vi "Add Item.vi"(7 "Action":T1, 8 "error in (no error)":errorcluster, 11 "Listbox Refs in":T2 {"Section Ref" format="%.0x"}) -> (0 "error out":errorcluster, 3 "Listbox Refs out":T2 {"Section Ref" format="%.0x"})   [LabVIEW 2016, in "FPGA Addon System Explorer.lvlib"]
uses:
  FPGA Addon System Explorer.lvlib
  Listbox Cluster.ctl
  <vilib>/NI Veristand/Custom Device API/Custom Device Item Ref.ctl
  FPGA-Resource-Manager-APIs/Source/Shared/Types/Channel Type.ctl
  <vilib>/NI Veristand/Custom Device API/Custom Device Channel.ctl
  <vilib>/NI Veristand/Custom Device API/Custom Device Channel Type.ctl
  FPGA/Speciality IO/Types/PWM.Measure.Analog.Settings.ctl
  FPGA/Speciality IO/Types/PWM.Generate.Digital.Settings.ctl
  FPGA/Speciality IO/Types/PWM.Generate.Digital.Convert.Settings.ctl
  FPGA/Speciality IO/Types/Sine.Generate.Settings.ctl
  FPGA/Speciality IO/Types/Sine.Generate.Convert.Settings.ctl
  FPGA/Speciality IO/Types/PWM.Measure.Digital.Settings.ctl
  FPGA/Speciality IO/Types/PWM.Measure.Analog.Result.ctl
  FPGA/Speciality IO/Types/PWM.Measure.Digital.Result.ctl
  FPGA-Resource-Manager-APIs/Source/System Definition/API/Server-Specific/Resource Groups/get fpga resources compatible with FPGA Addon CD group.vi
  Shared/Constants.vi
  RegMap to Register Information.vi
  FPGA-Resource-Manager-APIs/Source/System Definition/API/FPGA Resource Discovery/get FPGA resources for this FPGA Addon CD.vi
  FPGA-Resource-Manager-APIs/Source/Shared/find Relative VS Ref.vi
  <vilib>/NI Veristand/Custom Device API/NI VeriStand - Get Item Data.vi
  <vilib>/NI VeriStand/Custom Device API/Custom Device API.lvlib
  Shared/FPGA Addon Shared.lvlib
  FPGA/Speciality IO/Speciality FPGA IO.lvlib
  FPGA-Resource-Manager-APIs/Source/System Definition/FPGA RM System Definition API.lvlib
  FPGA-Resource-Manager-APIs/Source/Shared/FPGA RM Shared API.lvlib
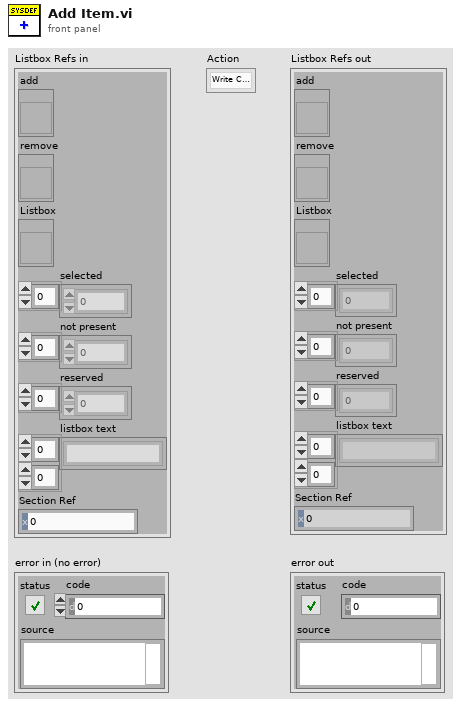
[diagram p1: front panel]
types:
  T1 = typedef "FPGA RM Shared API.lvlib/Channel Type.ctl" = enum16{"Write Channel", "Read Channel", "Write Waveform", "Read Waveform"}
  T2 = typedef "FPGA Addon System Explorer.lvlib/Listbox Cluster.ctl" = cluster{"add":refnum<vi>, "remove":refnum<vi>, "Listbox":refnum<vi>, "selected":i32[], "not present":i32[], "reserved":i32[], "listbox text":string[][], "Section Ref":T3}
  T3 = typedef "Custom Device API.lvlib/Custom Device Item Ref.ctl" = u64
  T4 = typedef "Custom Device API.lvlib/Custom Device Channel.ctl" = cluster{"Type":T5, "Units":string, "Default Value":dbl, "Faultable":bool, "Scalable":bool}
  T5 = typedef "Custom Device API.lvlib/Custom Device Channel Type.ctl" = enum16{"Input", "Output"}
  T6 = typedef "Speciality FPGA IO.lvlib/PWM.Measure.Analog.Settings.ctl" = cluster{"ACTIVE EDGE":bool, "TIMEOUT":u32, "THRESHOLD":fxp<+/-,32,8>}
  T7 = typedef "Speciality FPGA IO.lvlib/PWM.Generate.Digital.Convert.Settings.ctl" = cluster{"ACTIVE EDGE":bool, "FREQ":sgl, "DC":sgl}
  T8 = typedef "Speciality FPGA IO.lvlib/PWM.Generate.Digital.Settings.ctl" = cluster{"ACTIVE EDGE":bool, "ACTIVE TICKS":u32, "INACTIVE TICKS":u32}
  T9 = typedef "Speciality FPGA IO.lvlib/Sine.Generate.Convert.Settings.ctl" = cluster{"AMP":sgl, "OFFSET":sgl, "FREQ":sgl}
  T10 = typedef "Speciality FPGA IO.lvlib/Sine.Generate.Settings.ctl" = cluster{"AMP":fxp<+/-,32,8>, "OFFSET":fxp<+/-,32,8>, "PERIODS/TICKS":fxp<+,32,0>}
  T11 = typedef "Speciality FPGA IO.lvlib/PWM.Measure.Analog.Result.ctl" = cluster{"FREQ":sgl, "PERIOD":sgl, "DC":sgl, "ACTIVE TIME":sgl, "ACTIVE VOLTAGE":sgl, "INACTIVE VOLTAGE":sgl}
  T12 = typedef "Speciality FPGA IO.lvlib/PWM.Measure.Digital.Result.ctl" = cluster{"FREQ":sgl, "PERIOD":sgl, "DC":sgl, "ACTIVE TIME":sgl}
  T13 = typedef "FPGA RM Shared API.lvlib/Register Information.ctl" = cluster{"Name":string, "Data Type":T14, "Default Value":variant}
  T14 = typedef "FPGA RM Shared API.lvlib/Data Type.ctl" = enum8{"<Null>", "I8", "I16", "I32", "I64", "U8", "U16", "U32", "U64", "SGL", "Boolean", "Analog PWM In Settings", "Analog PWM In", "Digital PWM In Settings", "Digital PWM In", "Digital PWM Out", "Sine Out", "FXP+/-24.5", "FXP+/-16.5", "FXP+/-32.8", "FXP+/-64.32", "FXP+/-16.7", "FXP+/-20.5"}
  T15 = typedef "Speciality FPGA IO.lvlib/PWM.Measure.Digital.Settings.ctl" = cluster{"ACTIVE EDGE":bool, "TIMEOUT":u32}
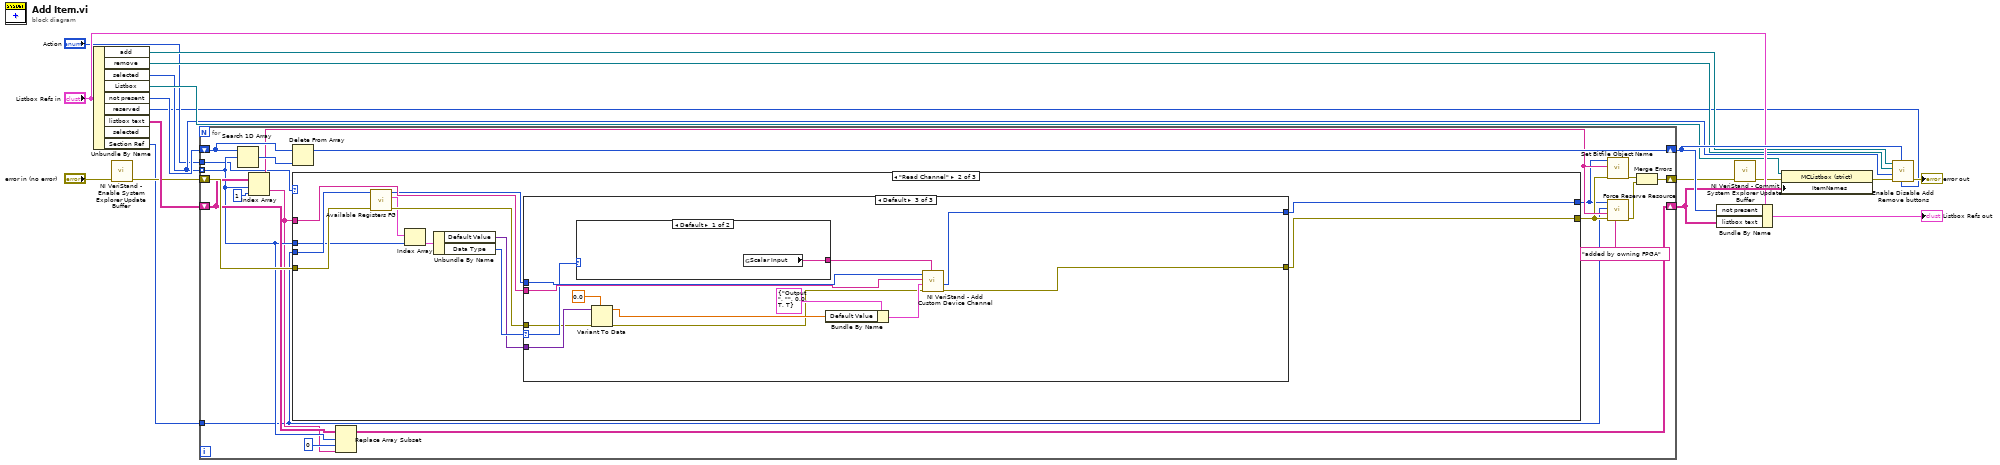
[diagram p0: block diagram]
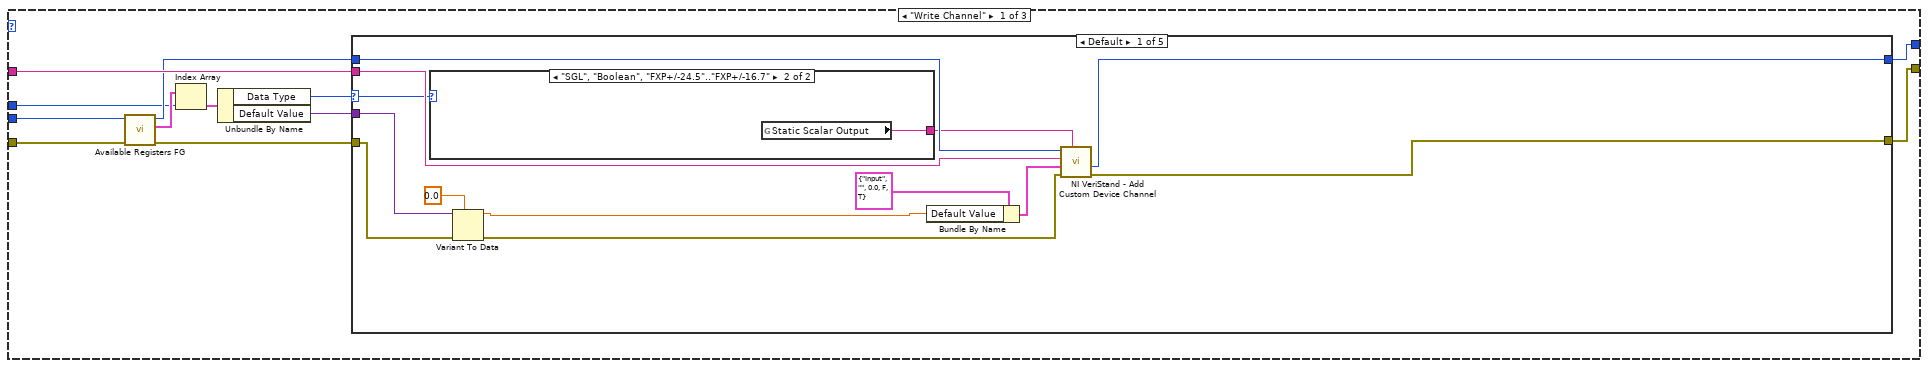
[diagram p2: hidden frame]
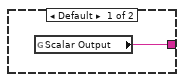
[diagram p3: hidden frame]
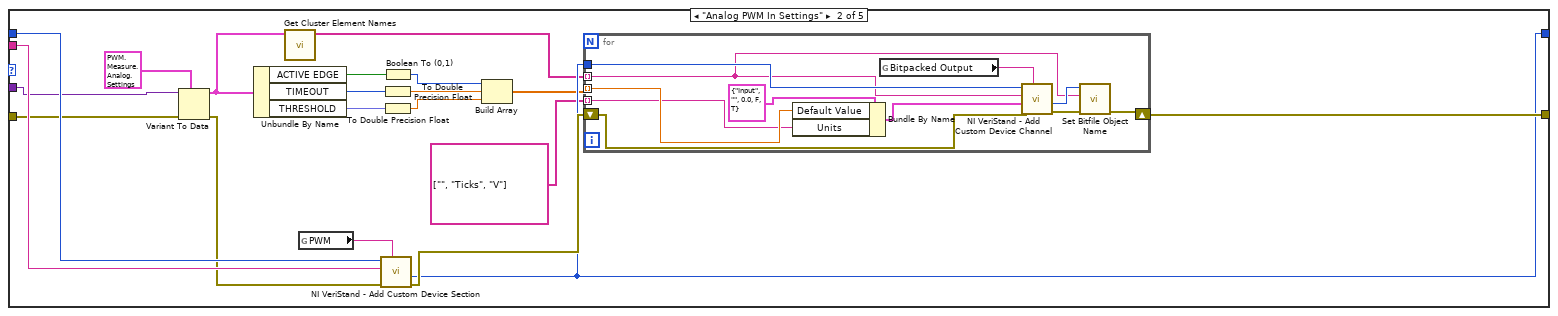
[diagram p4: hidden frame]
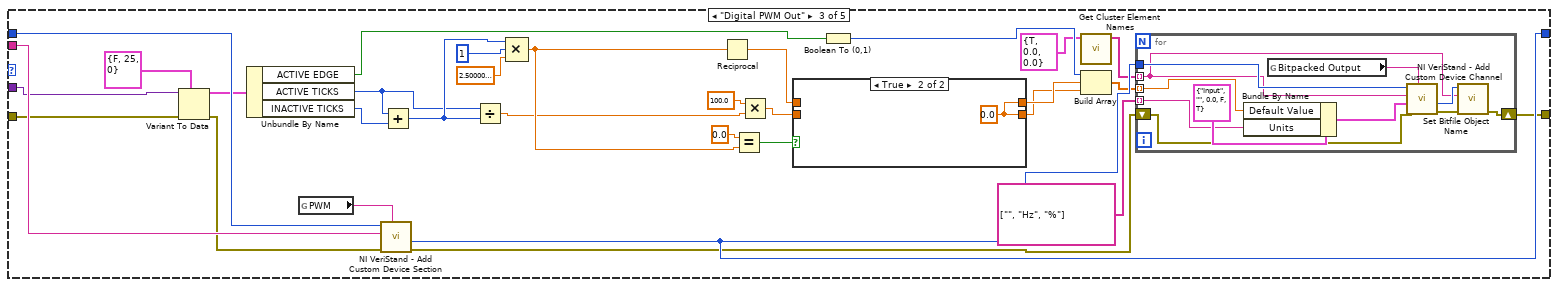
[diagram p5: hidden frame]
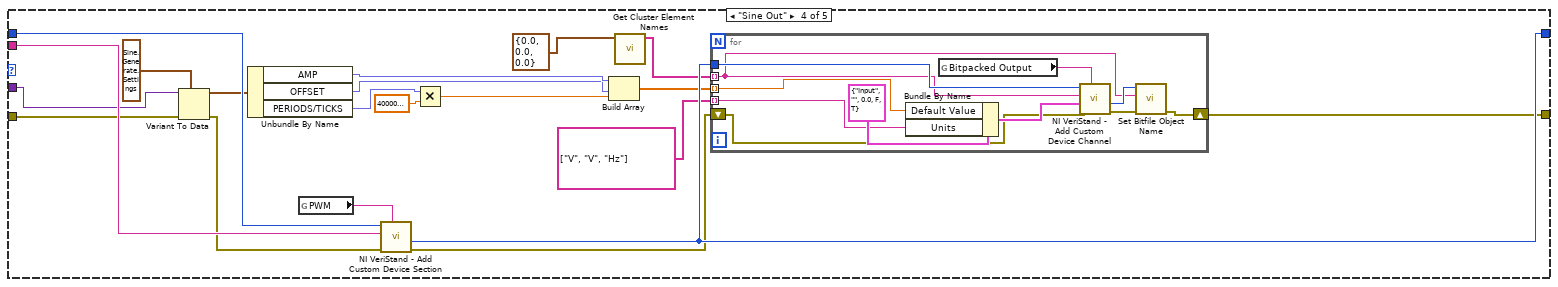
[diagram p7: hidden frame]
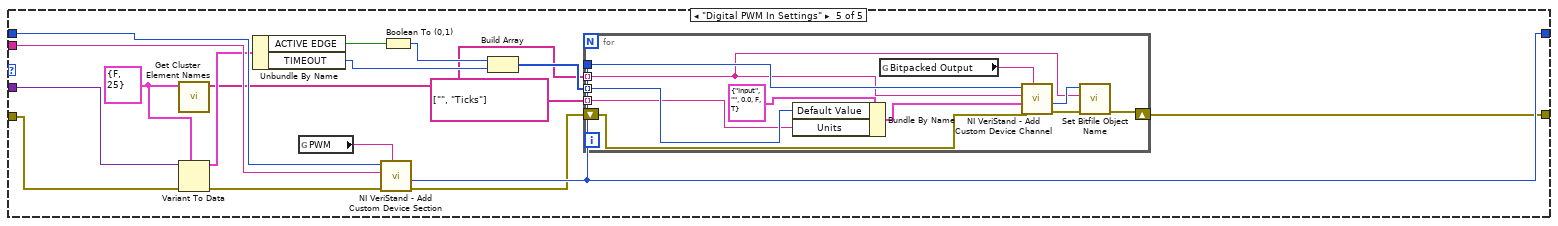
[diagram p8: hidden frame]
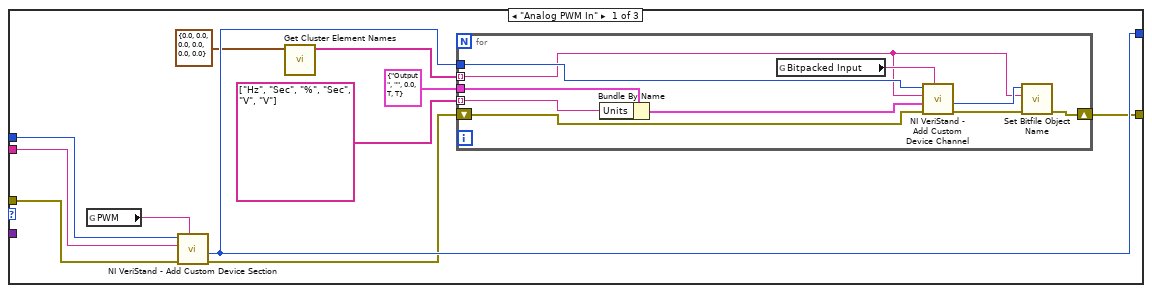
[diagram p9: hidden frame]
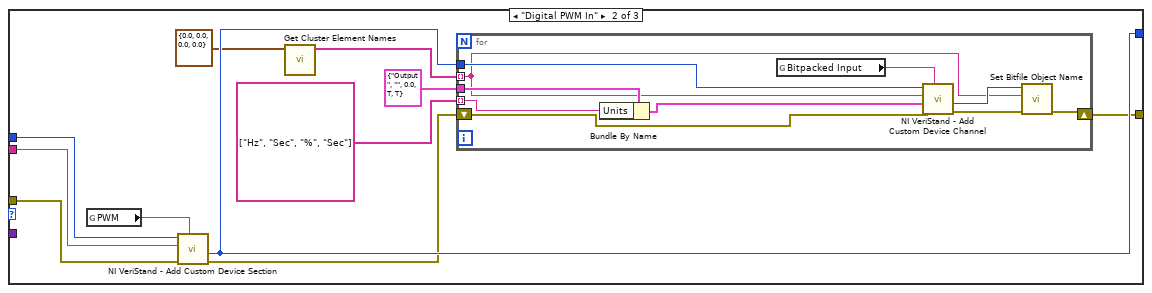
[diagram p10: hidden frame]
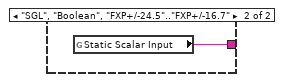
[diagram p11: hidden frame]
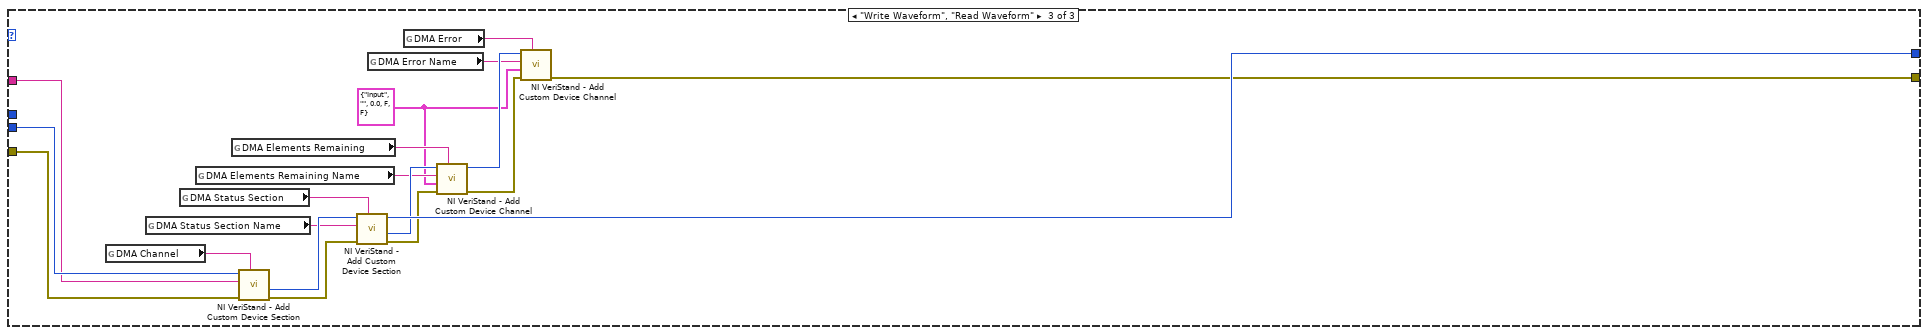
[diagram p12: hidden frame]
diagram:
  n1 = Unbundle By Name("Listbox Refs in") -> ("add"=w11:refnum<vi>, "remove"=w12:refnum<vi>, "selected"=w4:i32[], "Listbox"=w5:refnum<vi>, "not present"=w10:i32[], "reserved"=w1:i32[], "listbox text"=w18:string[][], "Section Ref"=w6:T3)  [unwired: 1 out]
  n2 = call <vilib>:"NI VeriStand - Enable System Explorer Update Buffer.vi"("error in (no error)"="error in (no error)") -> ("error out"=w9:errorcluster)  [unwired: 10 in]
  n3 = for {
    tunnel: w6 -> [w22]
    shift-right: [w25] -> w7
    shift-left: w9 -> [w37]
    tunnel: w4 -> [w29] mode=indexing
    shift-right: [w34] -> w16
    shift-left: w18 -> [w35]
    shift-right: [w30] -> w17
    shift-left: w10 -> [w32]
    tunnel: "Action" -> [w21]
    n4 = Search 1D Array(1D array=w32, element=w29) -> (index of element=w31:i32)  [unwired: 1 in]
    n5 = Index Array(array=w35, index (row)=w29, index (col)=1 ("disabled index (col)")) -> (element=w27:string)
    n6 = Delete From Array(array=w32, index=w31) -> (array with subset deleted=w30:i32[])  [unwired: 1 in, 1 out]
    n7 = case shown="\"Read Channel\"" w21 {
      tunnel: w37 -> [w44 w207 w286]
      tunnel: [w49 w211 w277] -> w26
      tunnel: w22 -> [w43 w208 w287]
      tunnel: w27 -> [w48 w210 w271]
      tunnel: [w47 w209 w282] -> w23
      tunnel: w29 -> [w40 w203 _]
      frame "Write Channel" {
        n8 = call "Available Registers FG.vi"("error in (no error)"=w44, "Item Ref"=w43) -> ("error out"=w41:errorcluster, "Available Registers"=w46:T13[], "Item Ref out"=w42:T3)  [unwired: 7 in]
        n9 = Index Array(array=w46, index=w40) -> (element=w45:T13)
        n10 = Unbundle By Name(w45) -> ("Data Type"=w38:T14, "Default Value"=w39:variant)
        n11 = case shown="Default" w38 {
          selector: w38 -> [w55 _ _ _ _]
          tunnel: [w62 w78 w120 w154 w182] -> w49
          tunnel: w48 -> [w61 w84 w126 w160 w188]
          tunnel: [w60 w77 w122 w156 w184] -> w47
          tunnel: w42 -> [w59 w83 w125 w159 w187]
          tunnel: w41 -> [w51 w81 w123 w157 w185]
          tunnel: w39 -> [w54 w82 w124 w158 w186]
          frame Default {
            n12 = case shown="\"SGL\", \"Boolean\", \"FXP+/-24.5\"..\"FXP+/-16.7\"" w55 {
              tunnel: [w63 w64] -> w58
              frame Default {
                n13 = global read "Constants.vi" "Scalar Output"() -> (w63:string)
              }
              frame "SGL", "Boolean", "FXP+/-24.5".."FXP+/-16.7" {
                n14 = global read "Constants.vi" "Static Scalar Output"() -> (w64:string)
              }
            }
            n15 = Variant To Data(error in=w51, type=0.0 ("Default Value"), Variant=w54) -> (data=w52:dbl, error out=w50:errorcluster)
            n16 = Bundle By Name(cluster=T4 {"Type"=enum."Input", "Units"="", "Default Value"=0.0, "Faultable"=FALSE, "Scalable"=TRUE} ("Channel"), "Default Value"=w52) -> (w56:T4)
            n17 = call <vilib>:"NI VeriStand - Add Custom Device Channel.vi"("GUID (Default Channel)"=w58, "error in (no error)"=w50, "Channel"=w56, "Channel Name"=w61, "Parent Ref in"=w59) -> ("error out"=w62:errorcluster, "Channel Ref"=w60:T3)  [unwired: 3 in, 2 out]
          }
          frame "Analog PWM In Settings" {
            n18 = Variant To Data(error in=w81, type=T6 {"ACTIVE EDGE"=FALSE, "TIMEOUT"=1000000000, "THRESHOLD"=25.0} ("Channel.Settings"), Variant=w82) -> (data=w66:T6, error out=w67:errorcluster)
            n19 = Unbundle By Name(w66) -> ("ACTIVE EDGE"=w72:bool, "TIMEOUT"=w76:u32, "THRESHOLD"=w71:fxp<+/-,32,8>)
            n20 = call "Get Cluster Element Names.vi"("Cluster"=w66) -> ("Channels"=w65:string[])  [unwired: 10 in]
            n21 = global read "Constants.vi" "PWM"() -> (w68:string)
            n22 = call <vilib>:"NI VeriStand - Add Custom Device Section.vi"("GUID (Default Section)"=w68, "error in (no error)"=w67, "Section Name"=w84, "Parent Ref in"=w83) -> ("error out"=w79:errorcluster, "Section Ptr"=w77:T3)  [unwired: 4 in, 2 out]
            n23 = Boolean To (0,1)(Boolean=w72) -> (0, 1=w70:i16)
            n24 = To Double Precision Float(number=w76) -> (double precision float=w74:dbl)
            n25 = To Double Precision Float(number=w71) -> (double precision float=w69:dbl)
            n26 = Build Array(w70, w74, w69) -> (w75:dbl[])
            n27 = for {
              tunnel: w77 -> [w93]
              shift-right: [w86] -> w78
              shift-left: w79 -> [w92]
              tunnel: w75 -> [w90] mode=indexing
              tunnel: string[] ["", "Ticks", "V"] -> [w89] mode=indexing
              tunnel: w65 -> [w85] mode=indexing
              n28 = Bundle By Name(cluster=T4 {"Type"=enum."Input", "Units"="", "Default Value"=0.0, "Faultable"=FALSE, "Scalable"=TRUE} ("Channel"), "Default Value"=w90, "Units"=w89) -> (w94:T4)
              n29 = global read "Constants.vi" "Bitpacked Output"() -> (w91:string)
              n30 = call <vilib>:"NI VeriStand - Add Custom Device Channel.vi"("GUID (Default Channel)"=w91, "error in (no error)"=w92, "Channel"=w94, "Channel Name"=w85, "Parent Ref in"=w93) -> ("error out"=w87:errorcluster, "Channel Ref"=w88:T3)  [unwired: 3 in, 2 out]
              n31 = call "Set Bitfile Object Name.vi"("error in (no error)"=w87, "Name"=w85, "Channel Ref"=w88) -> ("error out"=w86:errorcluster)  [unwired: 8 in]
            }
          }
          frame "Digital PWM Out" {
            n32 = Variant To Data(error in=w123, type=T8 {"ACTIVE EDGE"=FALSE, "ACTIVE TICKS"=25, "INACTIVE TICKS"=0} ("Channel.Settings"), Variant=w124) -> (data=w119:T8, error out=w112:errorcluster)
            n33 = Unbundle By Name(w119) -> ("ACTIVE EDGE"=w118:bool, "ACTIVE TICKS"=w103:u32, "INACTIVE TICKS"=w102:u32)
            n34 = global read "Constants.vi" "PWM"() -> (w115:string)
            n35 = call <vilib>:"NI VeriStand - Add Custom Device Section.vi"("GUID (Default Section)"=w115, "error in (no error)"=w112, "Section Name"=w126, "Parent Ref in"=w125) -> ("error out"=w121:errorcluster, "Section Ptr"=w122:T3)  [unwired: 4 in, 2 out]
            n36 = Add(x=w103, y=w102) -> (x+y=w109:u32)
            n37 = Divide(x=w103, y=w109) -> (x/y=w105:dbl)
            n38 = Compound Arithmetic op=MULTIPLY(w109, u32 1 ("value"), 2.5000000292152436e-08 ("y")) -> (w110:dbl)
            n39 = Reciprocal(x=w110) -> (1/x=w99:dbl)
            n40 = Equal?(x=0.0, y=w110) -> (x = y?=w101:bool)
            n41 = Multiply(x=100.0, y=w105) -> (x*y=w97:dbl)
            n42 = case shown="True" w101 {
              tunnel: [w128 w129] -> w100
              tunnel: w99 -> [w128 _]
              tunnel: [w127 w129] -> w98
              tunnel: w97 -> [w127 _]
              frame False {
              }
              frame True {
                w129 = 0.0
              }
            }
            n43 = Boolean To (0,1)(Boolean=w118) -> (0, 1=w117:i16)
            n44 = call "Get Cluster Element Names.vi"("Cluster"=T7 {"ACTIVE EDGE"=TRUE, "FREQ"=0.0, "DC"=0.0} ("Settings")) -> ("Channels"=w113:string[])  [unwired: 10 in]
            n45 = Build Array(w117, w100, w98) -> (w116:dbl[])
            n46 = for {
              tunnel: w122 -> [w138]
              shift-right: [w131] -> w120
              shift-left: w121 -> [w137]
              tunnel: w116 -> [w135] mode=indexing
              tunnel: w113 -> [w130] mode=indexing
              tunnel: string[] ["", "Hz", "%"] -> [w134] mode=indexing
              n47 = Bundle By Name(cluster=T4 {"Type"=enum."Input", "Units"="", "Default Value"=0.0, "Faultable"=FALSE, "Scalable"=TRUE} ("Channel"), "Default Value"=w135, "Units"=w134) -> (w139:T4)
              n48 = global read "Constants.vi" "Bitpacked Output"() -> (w136:string)
              n49 = call <vilib>:"NI VeriStand - Add Custom Device Channel.vi"("GUID (Default Channel)"=w136, "error in (no error)"=w137, "Channel"=w139, "Channel Name"=w130, "Parent Ref in"=w138) -> ("error out"=w132:errorcluster, "Channel Ref"=w133:T3)  [unwired: 3 in, 2 out]
              n50 = call "Set Bitfile Object Name.vi"("error in (no error)"=w132, "Name"=w130, "Channel Ref"=w133) -> ("error out"=w131:errorcluster)  [unwired: 8 in]
            }
          }
          frame "Sine Out" {
            n51 = Variant To Data(error in=w157, type=T10 {"AMP"=0.0, "OFFSET"=0.0, "PERIODS/TICKS"=0.0} ("Settings"), Variant=w158) -> (data=w153:T10, error out=w148:errorcluster)
            n52 = Unbundle By Name(w153) -> ("AMP"=w146:fxp<+/-,32,8>, "OFFSET"=w145:fxp<+/-,32,8>, "PERIODS/TICKS"=w144:fxp<+,32,0>)
            n53 = global read "Constants.vi" "PWM"() -> (w151:string)
            n54 = call <vilib>:"NI VeriStand - Add Custom Device Section.vi"("GUID (Default Section)"=w151, "error in (no error)"=w148, "Section Name"=w160, "Parent Ref in"=w159) -> ("error out"=w155:errorcluster, "Section Ptr"=w156:T3)  [unwired: 4 in, 2 out]
            n55 = Multiply(x=w144, y=sgl 40000000.0) -> (x*y=w142:sgl)
            n56 = Build Array(w146, w145, w142) -> (w152:sgl[])
            n57 = call "Get Cluster Element Names.vi"("Cluster"=T9 {"AMP"=0.0, "OFFSET"=0.0, "FREQ"=0.0} ("Settings")) -> ("Channels"=w149:string[])  [unwired: 10 in]
            n58 = for {
              tunnel: w156 -> [w169]
              shift-right: [w162] -> w154
              shift-left: w155 -> [w168]
              tunnel: w152 -> [w166] mode=indexing
              tunnel: w149 -> [w161] mode=indexing
              tunnel: string[] ["V", "V", "Hz"] -> [w165] mode=indexing
              n59 = Bundle By Name(cluster=T4 {"Type"=enum."Input", "Units"="", "Default Value"=0.0, "Faultable"=FALSE, "Scalable"=TRUE} ("Channel"), "Default Value"=w166, "Units"=w165) -> (w170:T4)
              n60 = global read "Constants.vi" "Bitpacked Output"() -> (w167:string)
              n61 = call <vilib>:"NI VeriStand - Add Custom Device Channel.vi"("GUID (Default Channel)"=w167, "error in (no error)"=w168, "Channel"=w170, "Channel Name"=w161, "Parent Ref in"=w169) -> ("error out"=w163:errorcluster, "Channel Ref"=w164:T3)  [unwired: 3 in, 2 out]
              n62 = call "Set Bitfile Object Name.vi"("error in (no error)"=w163, "Name"=w161, "Channel Ref"=w164) -> ("error out"=w162:errorcluster)  [unwired: 8 in]
            }
          }
          frame "Digital PWM In Settings" {
            w175 = T15 {"ACTIVE EDGE"=FALSE, "TIMEOUT"=25} ("Channel.Settings")
            n63 = call "Get Cluster Element Names.vi"("Cluster"=w175) -> ("Channels"=w174:string[])  [unwired: 10 in]
            n64 = Variant To Data(error in=w185, type=w175, Variant=w186) -> (data=w178:T15, error out=w173:errorcluster)
            n65 = Unbundle By Name(w178) -> ("ACTIVE EDGE"=w181:bool, "TIMEOUT"=w180:u32)
            n66 = global read "Constants.vi" "PWM"() -> (w176:string)
            n67 = call <vilib>:"NI VeriStand - Add Custom Device Section.vi"("GUID (Default Section)"=w176, "error in (no error)"=w173, "Section Name"=w188, "Parent Ref in"=w187) -> ("error out"=w183:errorcluster, "Section Ptr"=w184:T3)  [unwired: 4 in, 2 out]
            n68 = Boolean To (0,1)(Boolean=w181) -> (0, 1=w179:i16)
            n69 = Build Array(w179, w180) -> (w177:u32[])
            n70 = for {
              tunnel: w184 -> [w197]
              shift-right: [w191] -> w182
              shift-left: w183 -> [w196]
              tunnel: w177 -> [w194] mode=indexing
              tunnel: w174 -> [w189] mode=indexing
              tunnel: string[] ["", "Ticks"] -> [w193] mode=indexing
              n71 = Bundle By Name(cluster=T4 {"Type"=enum."Input", "Units"="", "Default Value"=0.0, "Faultable"=FALSE, "Scalable"=TRUE} ("Channel"), "Default Value"=w194, "Units"=w193) -> (w198:T4)
              n72 = global read "Constants.vi" "Bitpacked Output"() -> (w195:string)
              n73 = call <vilib>:"NI VeriStand - Add Custom Device Channel.vi"("GUID (Default Channel)"=w195, "error in (no error)"=w196, "Channel"=w198, "Channel Name"=w189, "Parent Ref in"=w197) -> ("error out"=w192:errorcluster, "Channel Ref"=w190:T3)  [unwired: 3 in, 2 out]
              n74 = call "Set Bitfile Object Name.vi"("error in (no error)"=w192, "Name"=w189, "Channel Ref"=w190) -> ("error out"=w191:errorcluster)  [unwired: 8 in]
            }
          }
        }
      }
      frame "Read Channel" {
        n75 = call "Available Registers FG.vi"("error in (no error)"=w207, "Item Ref"=w208) -> ("error out"=w206:errorcluster, "Available Registers"=w204:T13[], "Item Ref out"=w205:T3)  [unwired: 7 in]
        n76 = Index Array(array=w204, index=w203) -> (element=w202:T13)
        n77 = Unbundle By Name(w202) -> ("Default Value"=w200:variant, "Data Type"=w201:T14)
        n78 = case shown="Default" w201 {
          selector: w201 -> [_ _ w259]
          tunnel: [w217 w238 w266] -> w211
          tunnel: w210 -> [w220 w241 w265]
          tunnel: [w218 w239 w264] -> w209
          tunnel: w206 -> [w222 w243 w255]
          tunnel: w205 -> [w221 w242 w263]
          tunnel: w200 -> [_ _ w258]
          frame "Analog PWM In" {
            n79 = global read "Constants.vi" "PWM"() -> (w215:string)
            n80 = call <vilib>:"NI VeriStand - Add Custom Device Section.vi"("GUID (Default Section)"=w215, "error in (no error)"=w222, "Section Name"=w220, "Parent Ref in"=w221) -> ("error out"=w212:errorcluster, "Section Ptr"=w218:T3)  [unwired: 4 in, 2 out]
            n81 = call "Get Cluster Element Names.vi"("Cluster"=T11 {"FREQ"=0.0, "PERIOD"=0.0, "DC"=0.0, "ACTIVE TIME"=0.0, "ACTIVE VOLTAGE"=0.0, "INACTIVE VOLTAGE"=0.0} ("Analyzed")) -> ("Channels"=w213:string[])  [unwired: 10 in]
            n82 = for {
              tunnel: T4 {"Type"=enum."Output", "Units"="", "Default Value"=0.0, "Faultable"=TRUE, "Scalable"=TRUE} ("Channel") -> [w229]
              tunnel: w218 -> [w232]
              shift-right: [w224] -> w217
              shift-left: w212 -> [w231]
              tunnel: string[] ["Hz", "Sec", "%", "Sec", "V", "V"] -> [w227] mode=indexing
              tunnel: w213 -> [w223] mode=indexing
              n83 = Bundle By Name(cluster=w229, "Units"=w227) -> (w228:T4)
              n84 = global read "Constants.vi" "Bitpacked Input"() -> (w230:string)
              n85 = call <vilib>:"NI VeriStand - Add Custom Device Channel.vi"("GUID (Default Channel)"=w230, "error in (no error)"=w231, "Channel"=w228, "Channel Name"=w223, "Parent Ref in"=w232) -> ("error out"=w225:errorcluster, "Channel Ref"=w226:T3)  [unwired: 3 in, 2 out]
              n86 = call "Set Bitfile Object Name.vi"("error in (no error)"=w225, "Name"=w223, "Channel Ref"=w226) -> ("error out"=w224:errorcluster)  [unwired: 8 in]
            }
          }
          frame "Digital PWM In" {
            n87 = global read "Constants.vi" "PWM"() -> (w236:string)
            n88 = call <vilib>:"NI VeriStand - Add Custom Device Section.vi"("GUID (Default Section)"=w236, "error in (no error)"=w243, "Section Name"=w241, "Parent Ref in"=w242) -> ("error out"=w233:errorcluster, "Section Ptr"=w239:T3)  [unwired: 4 in, 2 out]
            n89 = call "Get Cluster Element Names.vi"("Cluster"=T12 {"FREQ"=0.0, "PERIOD"=0.0, "DC"=0.0, "ACTIVE TIME"=0.0} ("Analyzed")) -> ("Channels"=w234:string[])  [unwired: 10 in]
            n90 = for {
              tunnel: T4 {"Type"=enum."Output", "Units"="", "Default Value"=0.0, "Faultable"=TRUE, "Scalable"=TRUE} ("Channel") -> [w253]
              tunnel: w239 -> [w252]
              shift-right: [w244] -> w238
              shift-left: w233 -> [w251]
              tunnel: string[] ["Hz", "Sec", "%", "Sec"] -> [w248] mode=indexing
              tunnel: w234 -> [w246] mode=indexing
              n91 = Bundle By Name(cluster=w253, "Units"=w248) -> (w249:T4)
              n92 = global read "Constants.vi" "Bitpacked Input"() -> (w250:string)
              n93 = call <vilib>:"NI VeriStand - Add Custom Device Channel.vi"("GUID (Default Channel)"=w250, "error in (no error)"=w251, "Channel"=w249, "Channel Name"=w246, "Parent Ref in"=w252) -> ("error out"=w245:errorcluster, "Channel Ref"=w247:T3)  [unwired: 3 in, 2 out]
              n94 = call "Set Bitfile Object Name.vi"("error in (no error)"=w245, "Name"=w246, "Channel Ref"=w247) -> ("error out"=w244:errorcluster)  [unwired: 8 in]
            }
          }
          frame Default {
            n95 = case shown="Default" w259 {
              tunnel: [w267 w268] -> w262
              frame Default {
                n96 = global read "Constants.vi" "Scalar Input"() -> (w267:string)
              }
              frame "SGL", "Boolean", "FXP+/-24.5".."FXP+/-16.7" {
                n97 = global read "Constants.vi" "Static Scalar Input"() -> (w268:string)
              }
            }
            n98 = Variant To Data(error in=w255, type=0.0, Variant=w258) -> (data=w256:dbl, error out=w254:errorcluster)
            n99 = Bundle By Name(cluster=T4 {"Type"=enum."Output", "Units"="", "Default Value"=0.0, "Faultable"=TRUE, "Scalable"=TRUE} ("Channel"), "Default Value"=w256) -> (w260:T4)
            n100 = call <vilib>:"NI VeriStand - Add Custom Device Channel.vi"("GUID (Default Channel)"=w262, "error in (no error)"=w254, "Channel"=w260, "Channel Name"=w265, "Parent Ref in"=w263) -> ("error out"=w266:errorcluster, "Channel Ref"=w264:T3)  [unwired: 3 in, 2 out]
          }
        }
      }
      frame "Write Waveform", "Read Waveform" {
        w272 = T4 {"Type"=enum."Input", "Units"="", "Default Value"=0.0, "Faultable"=FALSE, "Scalable"=FALSE} ("Channel")
        n101 = global read "Constants.vi" "DMA Channel"() -> (w285:string)
        n102 = global read "Constants.vi" "DMA Status Section Name"() -> (w270:string)
        n103 = global read "Constants.vi" "DMA Status Section"() -> (w269:string)
        n104 = global read "Constants.vi" "DMA Elements Remaining Name"() -> (w275:string)
        n105 = global read "Constants.vi" "DMA Elements Remaining"() -> (w276:string)
        n106 = call <vilib>:"NI VeriStand - Add Custom Device Section.vi"("GUID (Default Section)"=w285, "error in (no error)"=w286, "Section Name"=w271, "Parent Ref in"=w287) -> ("error out"=w284:errorcluster, "Section Ptr"=w283:T3)  [unwired: 4 in, 2 out]
        n107 = call <vilib>:"NI VeriStand - Add Custom Device Section.vi"("GUID (Default Section)"=w269, "error in (no error)"=w284, "Section Name"=w270, "Parent Ref in"=w283) -> ("error out"=w278:errorcluster, "Section Ptr"=w279:T3, "Parent Ref out"=w282:T3)  [unwired: 4 in, 1 out]
        n108 = global read "Constants.vi" "DMA Error Name"() -> (w274:string)
        n109 = global read "Constants.vi" "DMA Error"() -> (w273:string)
        n110 = call <vilib>:"NI VeriStand - Add Custom Device Channel.vi"("GUID (Default Channel)"=w276, "error in (no error)"=w278, "Channel"=w272, "Channel Name"=w275, "Parent Ref in"=w279) -> ("error out"=w280:errorcluster, "Parent Ref out"=w281:T3)  [unwired: 3 in, 2 out]
        n111 = call <vilib>:"NI VeriStand - Add Custom Device Channel.vi"("GUID (Default Channel)"=w273, "error in (no error)"=w280, "Channel"=w272, "Channel Name"=w274, "Parent Ref in"=w281) -> ("error out"=w277:errorcluster)  [unwired: 3 in, 3 out]
      }
    }
    n112 = Replace Array Subset(array=w35, new element=w27, index (row)=w29, index (col)=0 ("disabled index (col)")) -> (w34:string[][])
    n113 = call "Set Bitfile Object Name.vi"("error in (no error)"=w26, "Name"=w27, "Channel Ref"=w23) -> ("error out"=w28:errorcluster)  [unwired: 8 in]
    n114 = call "Force Reserve Resource.vi"("notes"="added by owning FPGA", "error in (no error)"=w26, "Name in bitfile"=w27, "Client Node Ref"=w22, "Item Ref in"=w23) -> ("error out"=w24:errorcluster)  [unwired: 5 in, 1 out]
    n115 = Merge Errors(w28, w24) -> (w25:errorcluster)
  }
  n116 = Bundle By Name(cluster="Listbox Refs in", "not present"=w17, "listbox text"=w16) -> (→"Listbox Refs out":T2)
  n117 = call <vilib>:"NI VeriStand - Commit System Explorer Update Buffer.vi"("error in (no error)"=w7) -> ("error out"=w14:errorcluster)  [unwired: 10 in]
  n118 = property class="MCListbox (strict)"(reference=w5, error in=w14, "ItemNames"=w16) -> (error out=w13:errorcluster)  [unwired: 1 out]
  n119 = call "Enable Disable Add Remove buttons.vi"("reserved item indexes"=w1, "not present item indexes"=w17, "error in (no error)"=w13, "selected items"=w4, "remove button"=w12, "add button"=w11) -> ("error out"=→"error out":errorcluster)  [unwired: 5 in]
